vi "Parse Readings 6514.vi"(11 "Readings":string) -> (2 "Measurement":T1 {"Measurement" format="%.6e"}, 3 "Remain Readings":string)   [LabVIEW 2017, in "Keithley 6517.lvlib"]
doc: "Parse the readings according to the 6514 model format."
uses:
  Keithley 6517.lvlib
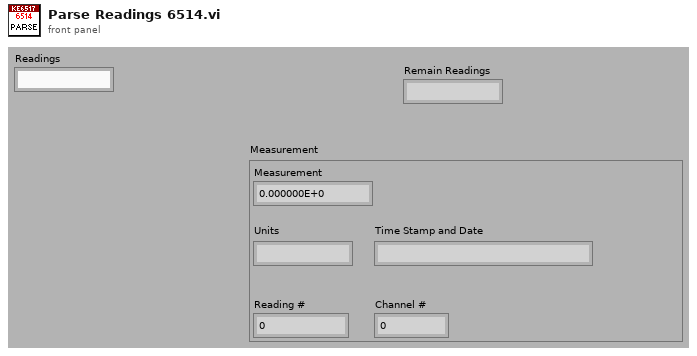
[diagram p1: front panel]
types:
  T1 = cluster{"Measurement":dbl, "Units":string, "Time Stamp and Date":string, "Reading #":dbl, "Channel #":dbl}
  T2 = cluster{dbl, string, "Readings":string, dbl, dbl}
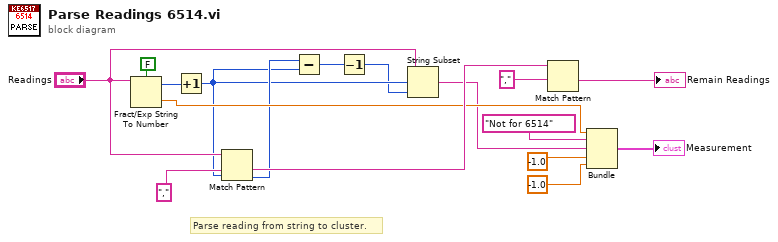
[diagram p0: block diagram]
diagram:
  # "Parse reading from string to cluster."
  n1 = Fract/Exp String To Number(use system decimal point (T)=FALSE, string="Readings") -> (offset past number=w10:i32, number=w13:dbl)  [unwired: 2 in]
  n2 = Increment(x=w10) -> (x+1=w3:i32)
  n3 = Match Pattern(string="Readings", regular expression=",", offset (0)=w3) -> (after substring=w15:string, offset past match=w8:i32)  [unwired: 2 out]
  n4 = Subtract(x=w8, y=w3) -> (x-y=w2:i32)
  n5 = Decrement(x=w2) -> (x-1=w1:i32)
  n6 = String Subset(string="Readings", offset (0)=w3, length (rest)=w1) -> (substring=w9:string)
  n7 = Match Pattern(string=w15, regular expression=",") -> (after substring=→"Remain Readings":string)  [unwired: 1 in, 3 out]
  n8 = Bundle(w13, "Not for 6514", "Readings"=w9, -1.0, -1.0) -> (→"Measurement":T2)  [unwired: 1 in]
